vi "Low Pass Differentiator - Heading.vi"(8 "Smoothing Factor":dbl=0.1, 10 "dt":dbl, 11 "Heading":T1 format="%05.1f") -> (3 "Heading Change, smoothed":dbl)   [LabVIEW 2011]
doc: "Differentiates the input and applies exponential smoothing to the output. Exponential smoothing weights the input value (in this case, the differentiated value) against the previous smoothing value."
uses:
  2 Typedefs/heading.ctl
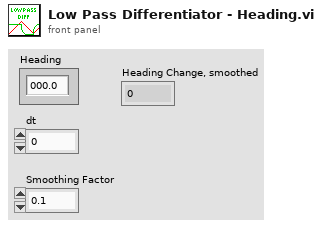
[diagram p1: front panel]
types:
  T1 = typedef "heading.ctl" = dbl
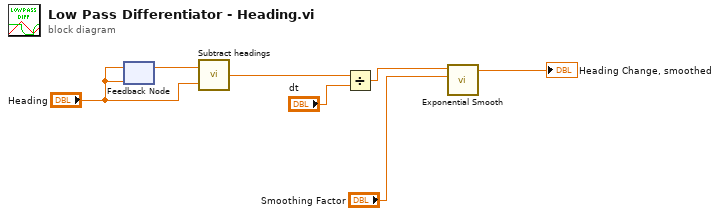
[diagram p0: block diagram]
diagram:
  n1 = feedback-in #1("Heading") -> ()
  n2 = feedback #1("Heading") -> (w1:T1)
  n3 = call "Subtract headings.vi"("Old Heading"="Heading", "New Heading"=w1) -> ("Heading Change"=w3:dbl)
  n4 = Divide(x=w3, y="dt") -> (x/y=w4:dbl)
  n5 = call "Exponential Smooth.vi"("Smoothing Factor"="Smoothing Factor", "Input Value"=w4) -> ("Smoothed Value"=→"Heading Change, smoothed":dbl)  [unwired: 9 in]
